vi "Record.vi"(8 "error in (no error)":errorcluster, 11 "Red Pitaya in":refnum<class "Red Pitaya.lvclass">) -> (0 "error out":errorcluster, 3 "Red Pitaya out":refnum<class "Red Pitaya.lvclass">)   [LabVIEW 2015, in "Red Pitaya.lvclass"]
uses:
  Red Pitaya.lvclass
  Red Pitaya.lvclass/Red Pitaya.ctl
  Red Pitaya Messages/Record Msg/Record Msg.lvclass
  <vilib>/ActorFramework/Actor/Actor.lvclass/Actor.ctl
  <vilib>/ActorFramework/Message Enqueuer/Message Enqueuer.lvclass/Message Enqueuer.ctl
  <vilib>/ActorFramework/Message Enqueuer/Init from Existing Queue.vi
  <vilib>/ActorFramework/Message Enqueuer/Message Enqueuer.lvclass
  <vilib>/ActorFramework/Actor/Actor.lvclass
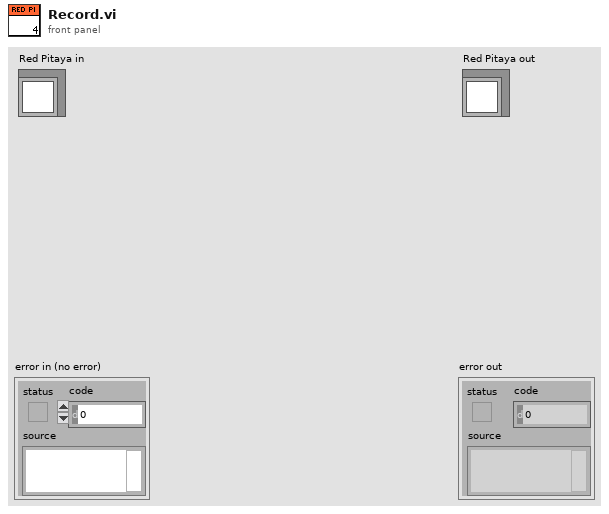
[diagram p1: front panel]
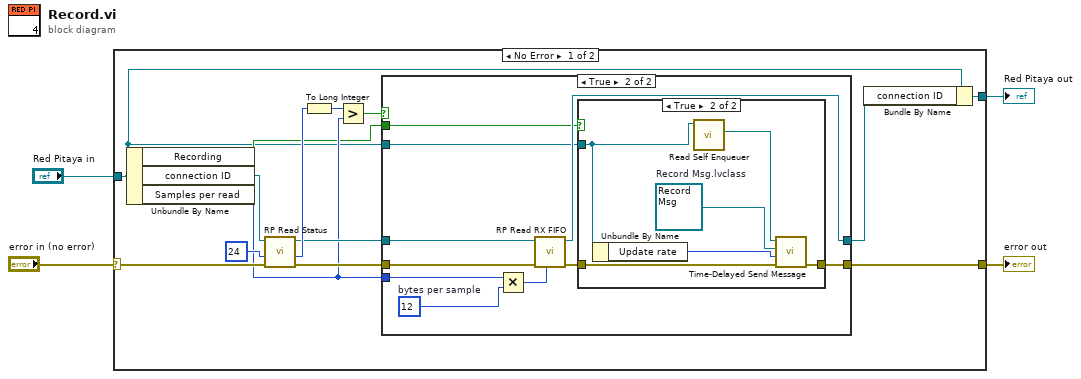
[diagram p0: block diagram]
diagram:
  n1 = case shown="No Error" "error in (no error)" {
    selector: "error in (no error)" -> [w18 w39]
    tunnel: [w9 w39] -> w3
    tunnel: [w8 w38] -> w1
    tunnel: "Red Pitaya in" -> [w5 w38]
    frame No Error {
      n2 = Unbundle By Name(w5) -> ("Recording"=w6:bool, "connection ID"=w12:refnum<k5>, "Samples per read"=w10:i32)
      n3 = call "RP Read Status.vi"("Error In"=w18, "Status offset"=u64 24, "connection ID"=w12) -> ("Error Out"=w13:errorcluster, "Status response"=w16:u32, "connection ID out"=w14:refnum<k5>)  [unwired: 6 in]
      n4 = To Long Integer(number=w16) -> (32bit integer=w11:i32)
      n5 = Greater?(x=w11, y=w10) -> (0:w15:bool)
      n6 = case shown="True" w15 {
        tunnel: w14 -> [w19 w30]
        tunnel: w13 -> [w20 w29]
        tunnel: w10 -> [_ w27]
        tunnel: [w20 w21] -> w9
        tunnel: [w19 w25] -> w7
        tunnel: w6 -> [_ w24]
        tunnel: w5 -> [_ w22]
        frame False {
        }
        frame True {
          w28 = 12  # bytes per sample
          n7 = Multiply(x=w27, y=w28) -> (x*y=w26:i32)
          n8 = call "RP Read RX FIFO.vi"("FIFO Bytes per read"=w26, "Error In"=w29, "connection ID"=w30) -> ("Error Out"=w23:errorcluster, "connection ID out"=w25:refnum<k5>)  [unwired: 4 in, 3 out]
          n9 = case shown="True" w24 {
            tunnel: w23 -> [w31 w37]
            tunnel: w22 -> [_ w35]
            tunnel: [w31 w33] -> w21
            frame False {
            }
            frame True {
              w34 = refnum<class "Record Msg.lvclass"> refnum  # Record Msg.lvclass
              n10 = Unbundle By Name(w35) -> ("Update rate"=w32:i32)
              n11 = call <vilib>:"Read Self Enqueuer.vi"("Actor"=w35) -> ("Self Enqueuer"=w36:refnum<class "Message Enqueuer.lvclass">)  [unwired: 10 in]
              n12 = call <vilib>:"Time-Delayed Send Message.vi"("error in (no error)"=w37, "Milliseconds To Wait"=w32, "Message"=w34, "Message Enqueuer"=w36) -> ("error out"=w33:errorcluster)  [unwired: 6 in, 1 out]
            }
          }
        }
      }
      n13 = Bundle By Name(cluster=w5, "connection ID"=w7) -> (w8:refnum<class "Red Pitaya.lvclass">)
    }
    frame Error {
    }
  }
  "error out" <- w3
  "Red Pitaya out" <- w1
